vi "DSF.Shared.Configuration.Plugin.Set Timing.vi"(10 "Timing":refnum<class "DSF.Shared.Timing.lvclass">, 11 "Plugin Configuration in":refnum<class "DSF.Shared.Configuration.Plugin.lvclass">) -> (3 "Plugin Configuration out":refnum<class "DSF.Shared.Configuration.Plugin.lvclass">)   [LabVIEW 2017, in "DSF.Shared.lvlib" / "DSF.Shared.Configuration.Plugin.lvclass"]
uses:
  DSF.Shared.Configuration.Plugin.lvclass
  Timing/DSF.Shared.Timing.lvclass
  DSF.Shared.Configuration.Plugin.lvclass/DSF.Shared.Configuration.Plugin.ctl
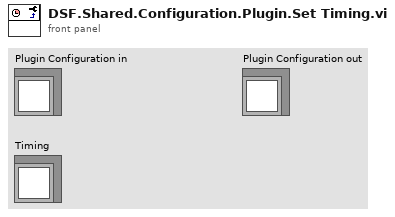
[diagram p1: front panel]
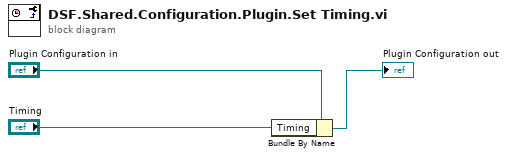
[diagram p0: block diagram]
diagram:
  n1 = Bundle By Name(cluster="Plugin Configuration in", "Timing"="Timing") -> (→"Plugin Configuration out":refnum<class "DSF.Shared.Configuration.Plugin.lvclass">)
